vi "test vi.vi"() -> (2 "Array 2":dbl[](array[numeric]))   [LabVIEW 2016]
panel:
  out "size(s) 2":i32[](array[numeric])
  out "array w/ subset deleted 2":i32[](array[numeric])
  out "deleted portion 2":i32[](array[numeric])
  in  "index 2":i32
  out "array w/ subset deleted":dbl[][](array[numeric])
  out "deleted portion":dbl[][](array[numeric])
  in  "disabled index (col) 2":i32
  in  "index (row) 2":i32
  in  "length":i32
  in  "delete array":bool
  out "x+y":dbl[](array[numeric])
  out "Array 3":i32[](array[numeric])
  in  "output array":dbl[][](array[numeric])
  out "element":dbl
  in  "disabled index (col)":i32
  in  "index (row)":i32
  out "size(s)":i32[](array[numeric])
  in  "new element/subarray 3":dbl[](array[numeric])
  out "s? t:f":dbl[][](array[numeric])
  in  "index":i32
  in  "start 2":bool
  in  "Array":dbl[](array[numeric])
  in  "stop":bool
  in  "start":bool
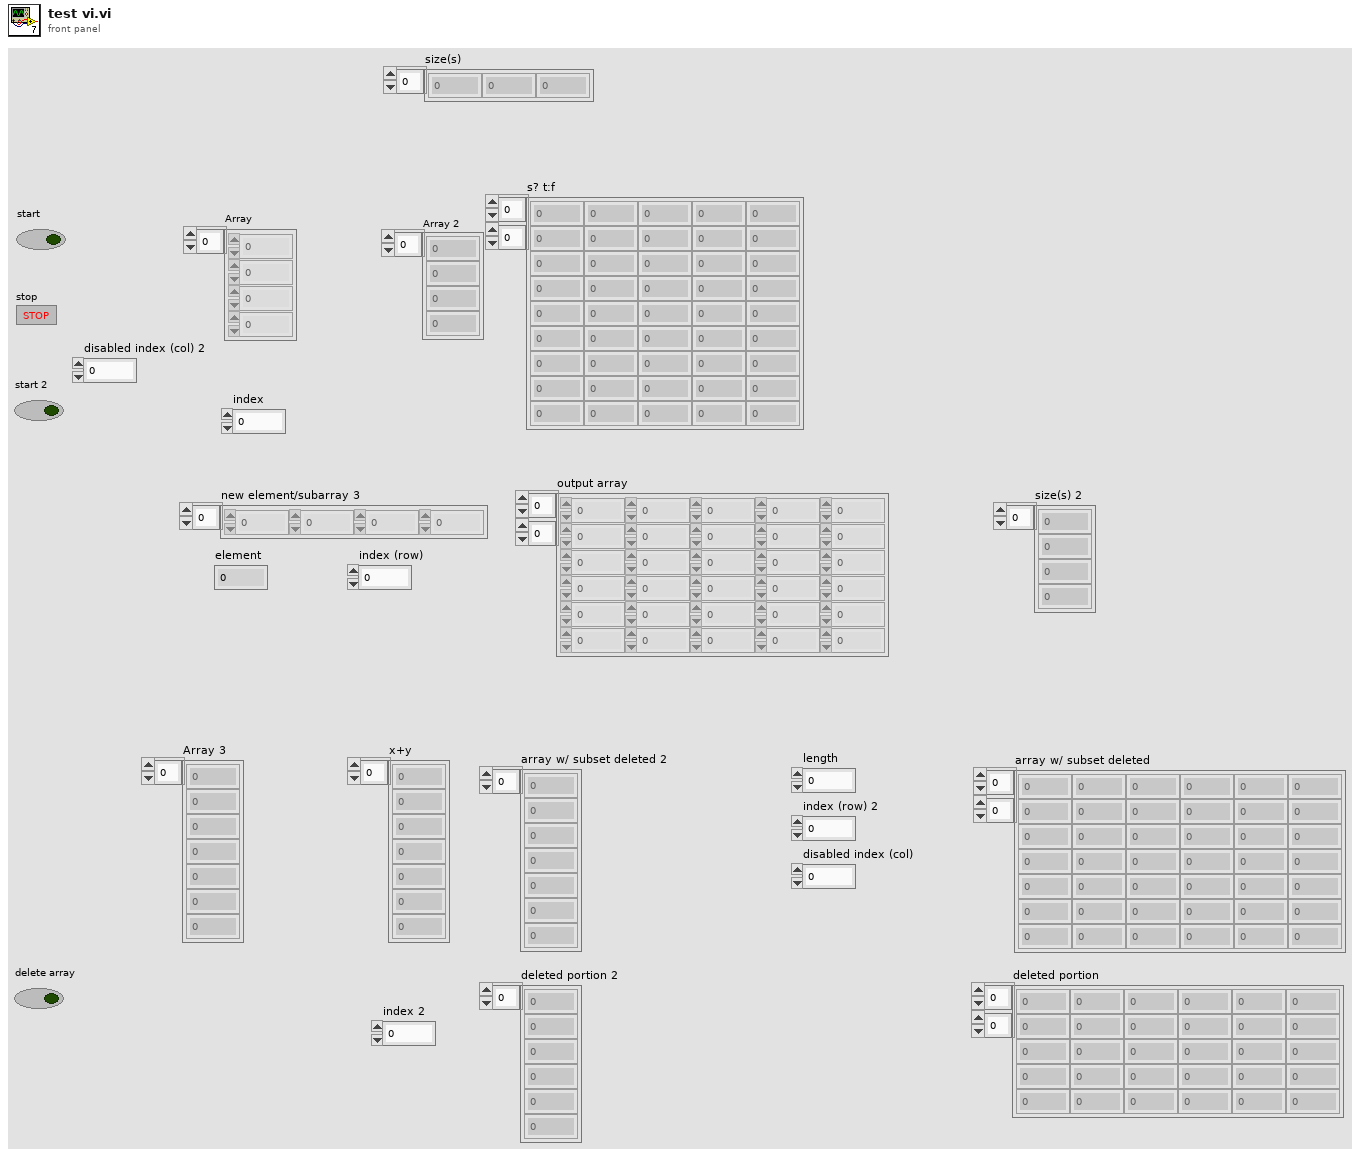
[diagram p1: front panel]
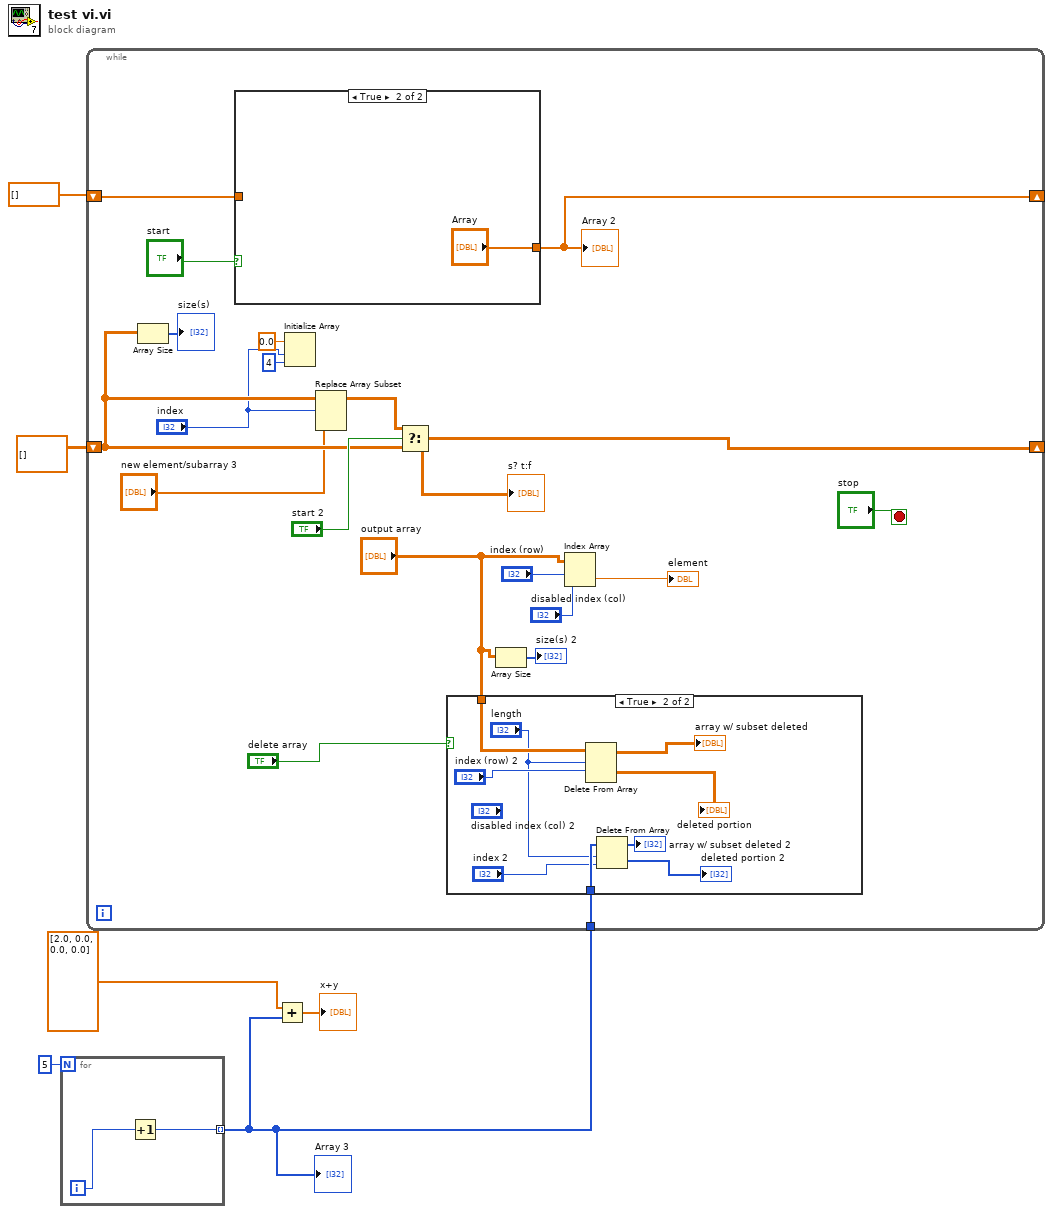
[diagram p0: block diagram]
diagram:
  n1 = for {
    N: 5 -> [_]
    tunnel: [w7] -> w1 mode=indexing
    i -> [w8]
    n2 = Increment(x=w8) -> (x+1=w7:i32)
  }
  "Array 3" <- w1
  n3 = while {
    shift-right: [w25] -> _
    shift-left: dbl[] [] ("Array") -> [w26]
    shift-right: [w24] -> _
    shift-left: dbl[][] [] ("Array") -> [w22]
    tunnel: w1 -> [w11]
    stop <- "stop" stop-if-true
    n4 = Array Size(array=w22) -> (size(s)=→"size(s)":i32[])
    n5 = case shown="True" "start" {
      tunnel: [w38 "Array"] -> w25
      tunnel: w26 -> [w38 _]
      frame False {
      }
      frame True {
      }
    }
    "Array 2" <- w25
    n6 = Initialize Array(0.0 ("element"), "index", 4 ("dimension size")) -> ()  [unwired: 1 out]
    n7 = Replace Array Subset(array=w22, new element="new element/subarray 3", index (row)="index") -> (w16:dbl[][])  [unwired: 1 in]
    n8 = Select(t=w16, s="start 2", f=w22) -> (s? t:f=w24:dbl[][])
    "s? t:f" <- w24
    n9 = case shown="True" "delete array" {
      tunnel: "output array" -> [_ w37]
      tunnel: w11 -> [_ w33]
      frame False {
      }
      frame True {
        n10 = Delete From Array(array=w37, length="length", index (row)="index (row) 2") -> (deleted portion=→"deleted portion":dbl[][], array with subset deleted=→"array w/ subset deleted":dbl[][])  [unwired: 1 in]
        n11 = Delete From Array(array=w33, length="length", index="index 2") -> (deleted portion=→"deleted portion 2":i32[], array with subset deleted=→"array w/ subset deleted 2":i32[])
      }
    }
    n12 = Array Size(array="output array") -> (size(s)=→"size(s) 2":i32[])
    n13 = Index Array(array="output array", index (row)="index (row)", index (col)="disabled index (col)") -> (element=→"element":dbl)
  }
  n14 = Add(x=dbl[] [2.0, 0.0, 0.0, 0.0] ("Array"), y=w1) -> (x+y=→"x+y":dbl[])
